vi "Terminate Condition Get Time At.vi"(4 "Minute Adder":dbl=1.0 format="%#_13g", 6 "Get Time At (Min)":dbl=24.0 format="%#_13g", 8 "error in":errorcluster, 10 "Normalized Timer Array in":dbl[](array[numeric]), 11 "Array in":dbl[][](array[numeric])) -> (0 "error out":errorcluster, 3 "Array out":dbl[][](array[numeric]))   [LabVIEW 2023]
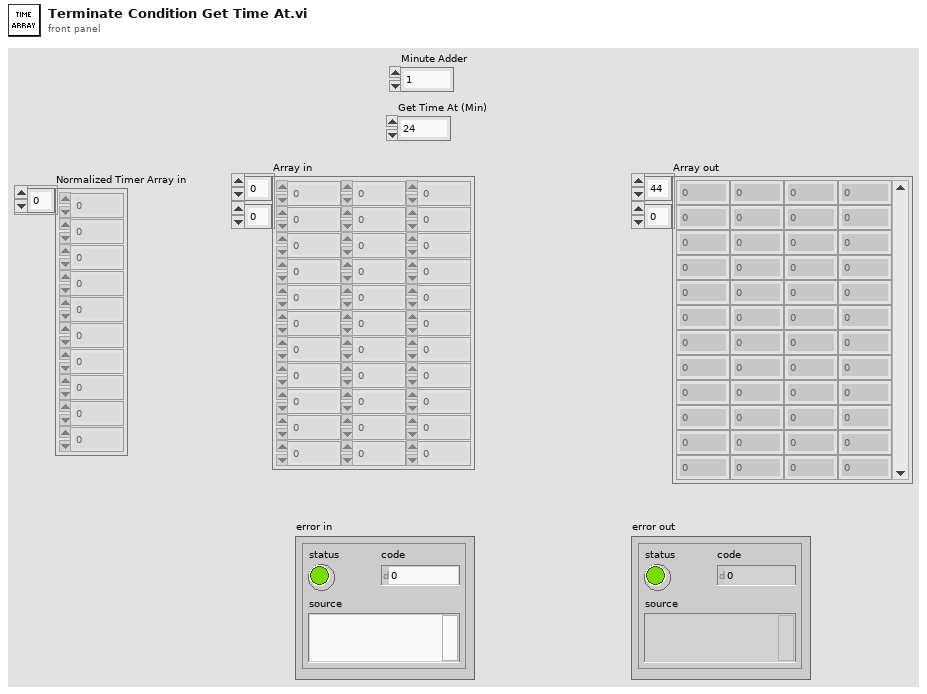
[diagram p1: front panel]
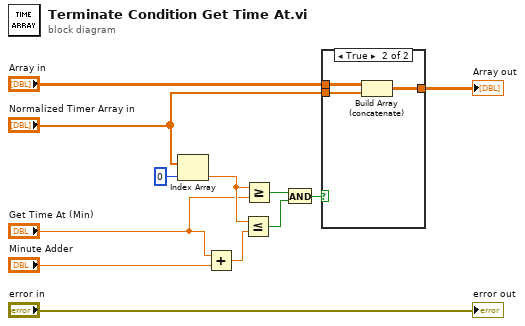
[diagram p0: block diagram]
diagram:
  n1 = Index Array(array="Normalized Timer Array in", index=0) -> (element=w6:dbl)
  n2 = Add(x="Get Time At (Min)", y="Minute Adder") -> (x+y=w4:dbl)
  n3 = Less Or Equal?(x=w6, y=w4) -> (x <= y?=w8:bool)
  n4 = Greater Or Equal?(x=w6, y="Get Time At (Min)") -> (x >= y?=w7:bool)
  n5 = And(x=w7, y=w8) -> (x .and. y?=w9:bool)
  n6 = case shown="True" w9 {
    tunnel: "Array in" -> [w13 w16]
    tunnel: "Normalized Timer Array in" -> [_ w15]
    tunnel: [w13 w14] -> w12
    frame False {
    }
    frame True {
      n7 = Build Array (concatenate)(w16, w15) -> (w14:dbl[][])
    }
  }
  "Array out" <- w12
  "error out" <- "error in"
